vi "Request Termination.vi"(8 "error in (no error)":errorcluster, 10 "force kill":bool, 11 "subprocess in":refnum<class "Buffered Subprocess.lvclass">) -> (0 "error out":errorcluster, 3 "subprocess out":refnum<class "Buffered Subprocess.lvclass">)   [LabVIEW 2020, in "NI_Subprocess.lvlib" / "Buffered Subprocess.lvclass"]
uses:
  <vilib>/Subprocess/Buffered Subprocess/Buffered Subprocess.lvclass
  <vilib>/Subprocess/Buffered Subprocess/Buffered Subprocess.lvclass/Buffered Subprocess.ctl
  <vilib>/Subprocess/Subprocess/Subprocess.lvclass
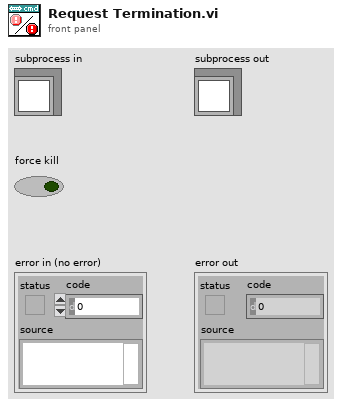
[diagram p1: front panel]
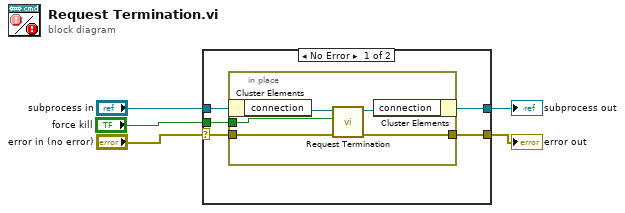
[diagram p0: block diagram]
diagram:
  n1 = case shown="No Error" "error in (no error)" {
    selector: "error in (no error)" -> [w9 w17]
    tunnel: [w8 w17] -> w4
    tunnel: [w7 w16] -> w2
    tunnel: "subprocess in" -> [w10 w16]
    tunnel: "force kill" -> [w6 _]
    frame No Error {
      n2 = in-place {
        in-place-border: w9 -> [w14]
        in-place-border: [w13] -> w8
        in-place-border: w6 -> [w11]
        n3 = in-place-cluster #1(w10) -> ("connection"=w15:refnum<class "Subprocess.lvclass">)
        n4 = call <vilib>:"Request Termination.vi"("error in (no error)"=w14, "force kill"=w11, "subprocess in"=w15) -> ("error out"=w13:errorcluster, "subprocess out"=w12:refnum<class "Subprocess.lvclass">)  [unwired: 7 in]
        n5 = in-place-cluster #1("connection"=w12) -> (w7:refnum<class "Buffered Subprocess.lvclass">)
      }
    }
    frame Error {
    }
  }
  "error out" <- w4
  "subprocess out" <- w2
